vi "DB_Update.vi"   [LabVIEW 2020]
uses:
  <vilib>/addons/database/Connection.llb/DB Tools Open Connec (String).vi
  <vilib>/addons/database/NI_Database_API.lvlib
types:
  T1 = typedef "NI_Database_API.lvlib/Conn ObjectReference.ctl" = refnum<k1>
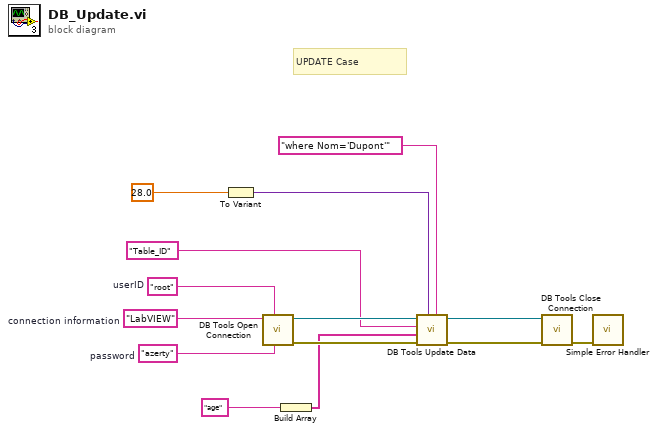
[diagram p0: block diagram]
diagram:
  w1 = "azerty"  # password
  w2 = "root"  # userID
  w3 = "LabVIEW"  # connection information
  # "UPDATE Case"
  n1 = To Variant(anything=sgl 28.0 ("age")) -> (Variant=w7:variant)
  n2 = call-poly <vilib>:"DB Tools Open Connection.vi"("password"=w1, "userID"=w2, "connection information"=w3) -> ("error out"=w13:errorcluster, "connection reference"=w14:T1)  [unwired: 5 in]
  n3 = Build Array("age" ("String")) -> (w9:string[])
  n4 = call <vilib>:"DB Tools Update Data.vi"("condition"="where Nom='Dupont'" ("format string"), "data"=w7, "error in (no error)"=w13, "columns"=w9, "table"="Table_ID", "connection reference"=w14) -> ("error out"=w4:errorcluster, "connection reference out"=w5:T1)  [unwired: 4 in]
  n5 = call <vilib>:"DB Tools Close Connection.vi"("error in (no error)"=w4, "connection reference"=w5) -> ("error out"=w12:errorcluster)  [unwired: 5 in]
  n6 = call <vilib>:"Simple Error Handler.vi"("error in (no error)"=w12) -> ()  [unwired: 4 in, 5 out]
